vi "gu_normalize_string.vi"(8 "error in":errorcluster, 10 "Normalized Form":T1, 11 "String":T2) -> (0 "error out":errorcluster, 3 "Normalized String":T2)   [LabVIEW 2020, in "G-Unicode.lvlib"]
uses:
  G-Unicode.lvlib
  lib/g_unicode_32.dll
  Types/Encoded UTF-8 String.ctl
  String/Controls/Normalized Form.ctl
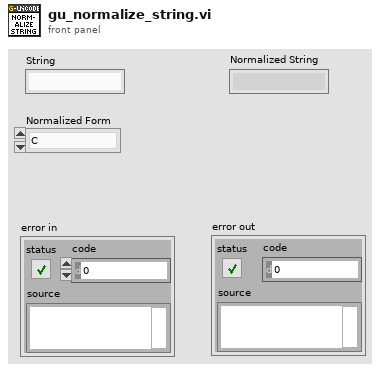
[diagram p1: front panel]
types:
  T1 = typedef "G-Unicode.lvlib/Normalized Form.ctl" = enum16{"C", "D", "KC", "KD"}
  T2 = typedef "G-Unicode.lvlib/Encoded UTF-8 String.ctl" = string
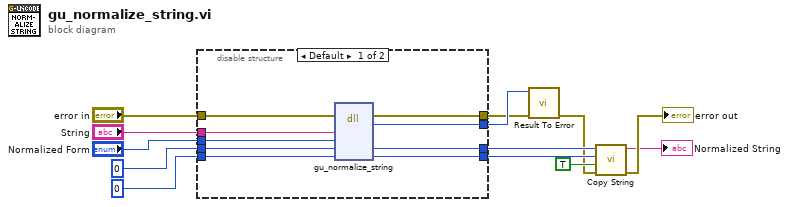
[diagram p0: block diagram]
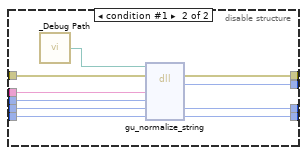
[diagram p2: hidden frame]
diagram:
  n1 = disable-structure shown="Default" {
    disable-tunnel: "String" -> [w21 w31]
    disable-tunnel: "error in" -> [w22 w32]
    disable-tunnel: [w18 w28] -> w3
    disable-tunnel: "Normalized Form" -> [w14 w23]
    disable-tunnel: 0 -> [w20 w30]
    disable-tunnel: i64 0 ("substring") -> [w19 w29]
    disable-tunnel: [w17 w27] -> w7
    disable-tunnel: [w16 w26] -> w6
    disable-tunnel: [w15 w24] -> w4
    frame condition #0 (active) {
      n2 = dll-call lib="C:/github/dataflowg/g-unicode/src/LabVIEW/G-Unicode/lib/g_unicode_*.*" fn="gu_normalize_string"(error in=w22, "string"=w21, "norm_form"=w14, "normalized"=w19, "normalized_size"=w20) -> (error out=w18:errorcluster, "result"=w15:i32, "normalized"=w17:i64, "normalized_size"=w16:i32)  [unwired: 4 in, 1 out]
    }
    frame condition #1 {
      n3 = call "_Debug Path.vi"() -> ("Debug Path"=w25:path)
      n4 = dll-call lib="?" fn="gu_normalize_string"(path in=w25, error in=w32, "string"=w31, "norm_form"=w23, "normalized"=w29, "normalized_size"=w30) -> (error out=w28:errorcluster, "result"=w24:i32, "normalized"=w27:i64, "normalized_size"=w26:i32)  [unwired: 3 in, 1 out]
    }
  }
  n5 = call "Result To Error.vi"("error in (no error)"=w3, "Result Code"=w4) -> ("error out"=w2:errorcluster)  [unwired: 9 in]
  n6 = call "Copy String.vi"("error in"=w2, "free (F)"=TRUE, "size"=w6, "pointer"=w7) -> ("error out"=→"error out":errorcluster, "string"=→"Normalized String":string)  [unwired: 6 in]
